vi "Joint Points FGV.vi"(6 "Command":T2(ring), 8 "error in (no error)":errorcluster, 9 "Body Index":i32, 10 "Joint Position":T1 {"TrackingState" items=["NotTracked", "Inferred", "Tracked"]}, 11 "name":string) -> (0 "error out":errorcluster, 2 "Joint Position":T1 {"TrackingState" items=["NotTracked", "Inferred", "Tracked"]})   [LabVIEW 2011, in "LVH-KinectOne.lvlib"]
uses:
  LVH-KinectOne.lvlib
  Type Defs/Joint Position.ctl
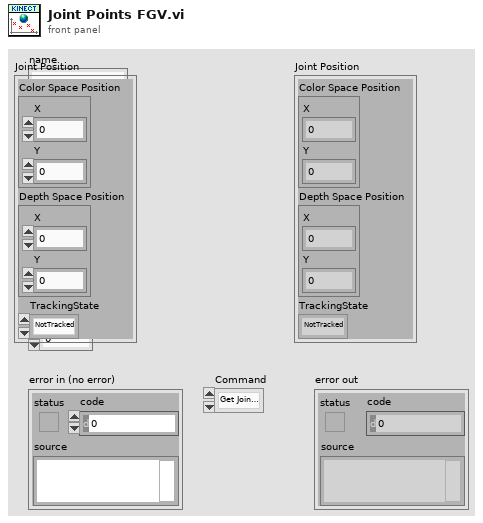
[diagram p1: front panel]
types:
  T1 = typedef "LVH-KinectOne.lvlib/Joint Position.ctl" = cluster{"Color Space Position":cluster{"X":sgl, "Y":sgl}, "Depth Space Position":cluster{"X":sgl, "Y":sgl}, "TrackingState":i32}
  T2 = enum16{"Get Joint Position", "Initialize", "Set Joint Position"}
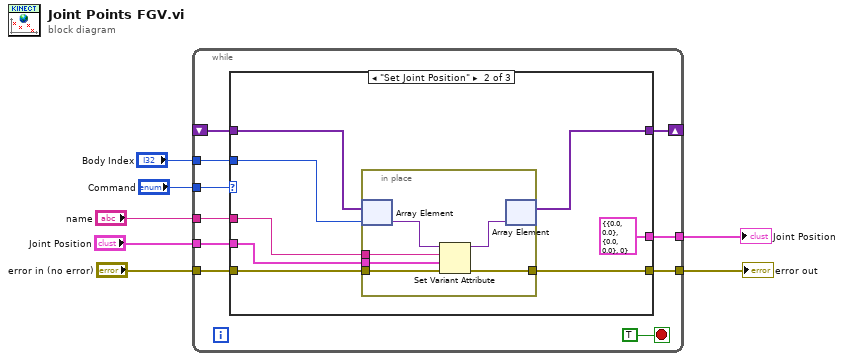
[diagram p0: block diagram]
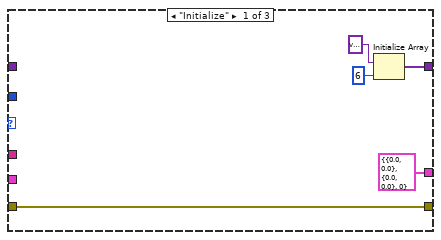
[diagram p2: hidden frame]
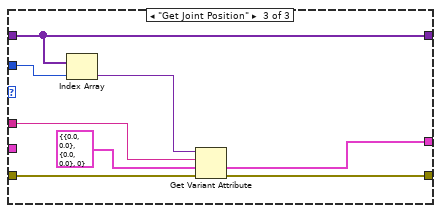
[diagram p3: hidden frame]
diagram:
  n1 = while {
    tunnel: "Command" -> [w16]
    shift-right: [w15] -> _
    shift-left: _ -> [w14]
    tunnel: "error in (no error)" -> [w13]
    tunnel: "name" -> [w12]
    tunnel: [w11] -> w4
    tunnel: "Joint Position" -> [w10]
    tunnel: [w9] -> w2
    tunnel: "Body Index" -> [w8]
    stop <- TRUE stop-if-true
    n2 = case shown="\"Set Joint Position\"" w16 {
      tunnel: [w18 w24 w39] -> w15
      tunnel: w14 -> [_ w26 w39]
      tunnel: w13 -> [w22 w30 w44]
      tunnel: w12 -> [_ w29 w43]
      tunnel: [w22 w28 w42] -> w11
      tunnel: w10 -> [_ w27 _]
      tunnel: [T1 {"Color Space Position"={"X"=0.0, "Y"=0.0}, "Depth Space Position"={"X"=0.0, "Y"=0.0}, "TrackingState"=0} ("Joint Position") T1 {"Color Space Position"={"X"=0.0, "Y"=0.0}, "Depth Space Position"={"X"=0.0, "Y"=0.0}, "TrackingState"=0} ("Joint Position") w41] -> w9
      tunnel: w8 -> [_ w25 w38]
      frame "Initialize" {
        n3 = Initialize Array(variant ("variant out"), 6 ("dimension size")) -> (w18:variant[])
      }
      frame "Set Joint Position" {
        n4 = in-place {
          in-place-border: w30 -> [w36]
          in-place-border: w29 -> [w35]
          in-place-border: [w34] -> w28
          in-place-border: w27 -> [w33]
          n5 = in-place-array #1(w26, w25) -> (w32:variant)
          n6 = Set Variant Attribute(Variant=w32, name=w35, value=w33, error in=w36) -> (Variant out=w31:variant, error out=w34:errorcluster)  [unwired: 1 out]
          n7 = in-place-array #1(w31) -> (w24:variant[])  [unwired: 1 out]
        }
      }
      frame "Get Joint Position" {
        n8 = Index Array(array=w39, index=w38) -> (element=w40:variant)
        n9 = Get Variant Attribute(Variant=w40, name=w43, default value (empty Variant)=T1 {"Color Space Position"={"X"=0.0, "Y"=0.0}, "Depth Space Position"={"X"=0.0, "Y"=0.0}, "TrackingState"=0} ("Joint Position"), error in=w44) -> (value=w41:T1, error out=w42:errorcluster)  [unwired: 2 out]
      }
    }
  }
  "error out" <- w4
  "Joint Position" <- w2
